vi "Match Exact String.vi"(1 "String":string, 4 "string array":string[](array[string])) -> (18 "index":i32)   [LabVIEW 2009, in "PTUtils.lvlib"]
uses:
  PTUtils.lvlib
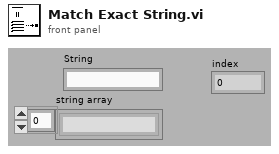
[diagram p1: front panel]
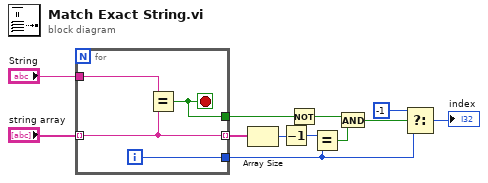
[diagram p0: block diagram]
diagram:
  n1 = for {
    tunnel: "string array" -> [w14] mode=indexing
    tunnel: "String" -> [w16]
    tunnel: [w15] -> w3
    tunnel: [w14] -> w10 mode=indexing
    tunnel: [w13] -> w7
    i -> [w15]
    stop <- w13 stop-if-true
    n2 = Equal?(x=w16, y=w14) -> (x = y?=w13:bool)
  }
  n3 = Array Size(array=w10) -> (size(s)=w9:i32)
  n4 = Decrement(x=w9) -> (x-1=w8:i32)
  n5 = Not(x=w7) -> (.not. x?=w6:bool)
  n6 = Equal?(x=w8, y=w3) -> (x = y?=w5:bool)
  n7 = And(x=w6, y=w5) -> (x .and. y?=w4:bool)
  n8 = Select(t=-1, s=w4, f=w3) -> (s? t:f=→"index":i32)
